vi "test.vi"(8 "error in (no error)":errorcluster, 11 "SPARC4_Channel in":refnum<class "SPARC4_Channel.lvclass">) -> (0 "error out":errorcluster, 2 "Sim_CCD.lvclass":refnum<class "Sim_CCD.lvclass">, 3 "SPARC4_Channel out":refnum<class "SPARC4_Channel.lvclass">)   [LabVIEW 2018, in "SPARC4_Channel.lvclass"]
uses:
  SPARC4_Channel.lvclass
  Sim_CCD/Sim_CCD.lvclass
  Sim_Ixon_Ultra/Sim_Ixon_Ultra.lvclass
  C:/Users/Denis/Desktop/S4ACS/S4ACS/Sim_CCD/Sim_CCD.lvclass
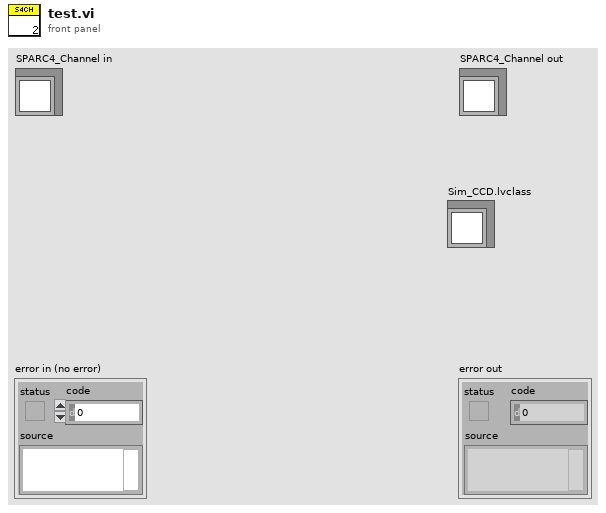
[diagram p1: front panel]
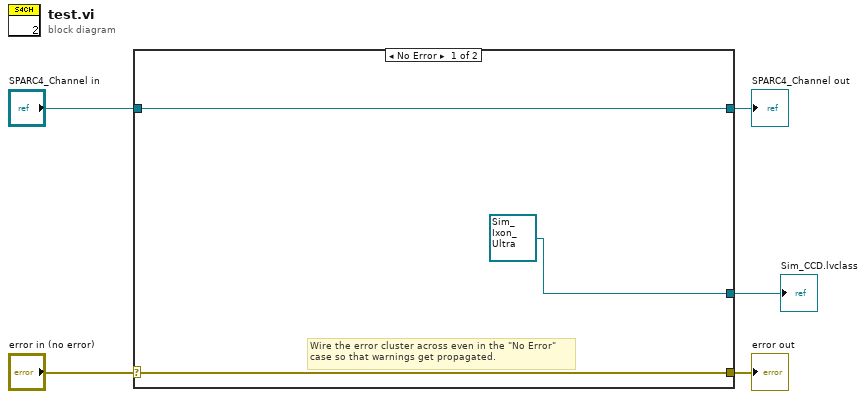
[diagram p0: block diagram]
diagram:
  n1 = case shown="No Error" "error in (no error)" {
    selector: "error in (no error)" -> [w7 w10]
    tunnel: [w7 w10] -> w4
    tunnel: [w8 w9] -> w2
    tunnel: "SPARC4_Channel in" -> [w8 w9]
    tunnel: [refnum<class "Sim_Ixon_Ultra.lvclass"> refnum ("Sim_Ixon_Ultra.lvclass") _] -> w1
    frame No Error {
      # "Wire the error cluster across even in the \"No Error\"\ncase so that warnings get propagated."
    }
    frame Error {
    }
  }
  "error out" <- w4
  "SPARC4_Channel out" <- w2
  "Sim_CCD.lvclass" <- w1
